vi "TCP lesen - Amium.vi"(6 "Timeout":i32=80, 8 "Fehler (Eingang)":errorcluster caption="Fehler (Eingang, kein Fehler)", 11 "connection ID":refnum<k5>) -> (0 "error out":errorcluster, 2 "Daten (Ausgang)":string, 3 "connection ID":refnum<k5>)   [LabVIEW 2020, in "Amium PNS.lvlib" / "AK Kommunikation.lvlib"]
uses:
  AK Kommunikation.lvlib
panel:
  # "Ablaufinvariante Ausführung"
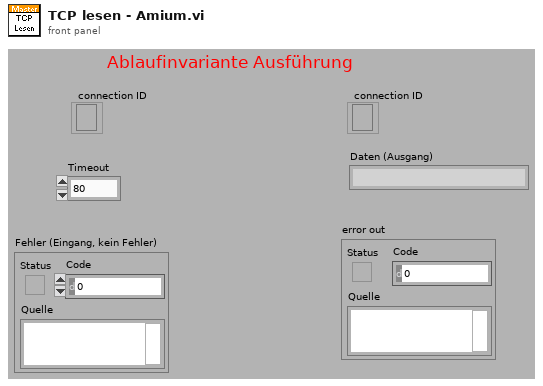
[diagram p1: front panel]
types:
  T1 = enum16{"Standard", "Buffered", "CRLF", "Immediate"}
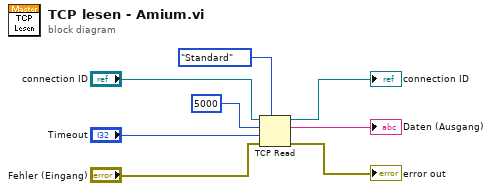
[diagram p0: block diagram]
diagram:
  n1 = TCP Read(connection ID="connection ID", bytes to read=5000 ("Zu lesende Bytes"), error in (no error)="Fehler (Eingang)", 7:T1."Standard" ("Modus (Standard)"), 9:"Timeout") -> (connection ID out=→"connection ID":refnum<k5>, data out=→"Daten (Ausgang)":string, error out=→"error out":errorcluster)
